vi "Get Parent Libraries.vi"(8 "error in (no error)":errorcluster {"code" format="Error %.0f"}, 11 "Class Documentation In":refnum<class "Class Documentation.lvclass">) -> (0 "error out":errorcluster {"code" format="Error %.0f"}, 2 "Parent Libraries":T1[](array[typedef]), 3 "Class Documentation Out":refnum<class "Class Documentation.lvclass">)   [LabVIEW 2023, in "VIDoc Parsing.lvlib" / "Class Documentation.lvclass"]
uses:
  Class Documentation.lvclass
  <vilib>/Utility/miscctls.llb/NI.Parent Library Information.ctl
  <vilib>/Utility/miscctls.llb/NI.Parent Library Kind.ctl
  Class Documentation.lvclass/Class Documentation.ctl
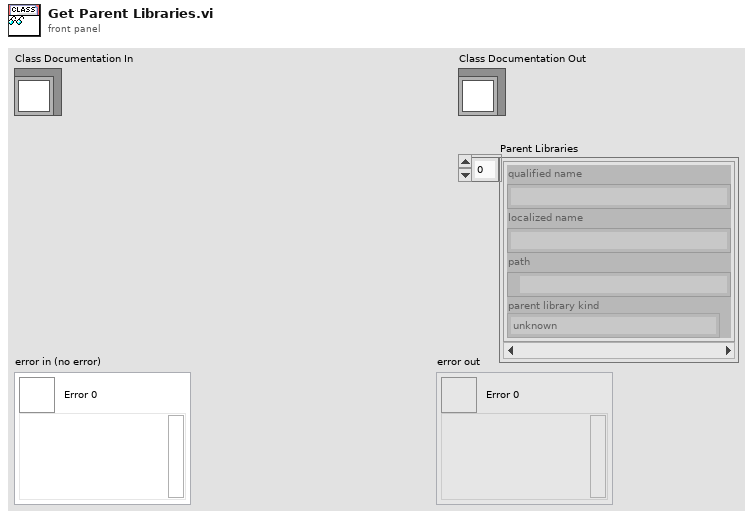
[diagram p1: front panel]
types:
  T1 = typedef "NI.Parent Library Information.ctl" = cluster{"qualified name":string, "localized name":string, "path":path, "parent library kind":T2}
  T2 = typedef "NI.Parent Library Kind.ctl" = enum32{"unknown", "class", "interface"}
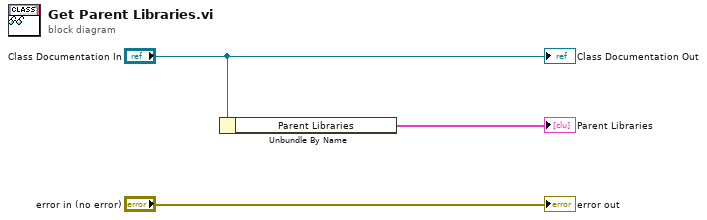
[diagram p0: block diagram]
diagram:
  n1 = Unbundle By Name("Class Documentation In") -> ("Parent Libraries"=→"Parent Libraries":T1[])
  "error out" <- "error in (no error)"
  "Class Documentation Out" <- "Class Documentation In"
